vi "Drive States.vi"(10 "Drive Metrics in":T1) -> (2 "Drive Metrics out":T1)   [LabVIEW 2014]
uses:
  Drive Metrics.ctl
  Drive States.ctl
  Global Objects.vi
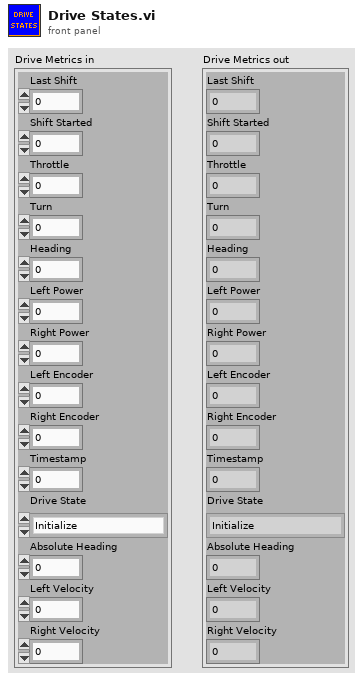
[diagram p1: front panel]
types:
  T1 = typedef "Drive Metrics.ctl" = cluster{"Last Shift":u32, "Shift Started":u32, "Throttle":dbl, "Turn":dbl, "Heading":dbl, "Left Power":dbl, "Right Power":dbl, "Left Encoder":dbl, "Right Encoder":dbl, "Timestamp":dbl, "Drive State":T2, "Absolute Heading":dbl, "Left Velocity":dbl, "Right Velocity":dbl}
  T2 = typedef "Drive States.ctl" = enum16{"Initialize", "Low Gear", "Up Shift Begin", "Up Shifting", "Up Shift Delay", "High Gear", "Down Shift Begin", "Down Shifting", "Down Shift Delay"}
  T3 = typedef "Configuration.ctl" = cluster{"Throttle Dead Zone":dbl, "Throttle Ramp Rate":dbl, "Turn Dead Zone":dbl, "Auton":cluster{"Motion Plan P":dbl, "Motion Plan I":dbl, "Motion Plan D":dbl}, "Auto Upshift Enabled":bool, "Upshift Min Throttle":dbl, "Upshift Min Velocity":dbl, "Min time before upshift":dbl, "Shift Throttle Detent":u32, "Min time before downshift":dbl, "Turn PID":cluster{"Motion Plan P":dbl, "Motion Plan I":dbl, "Motion Plan D":dbl}}
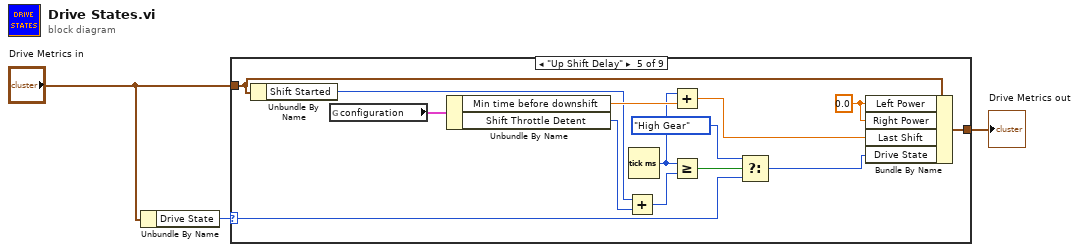
[diagram p0: block diagram]
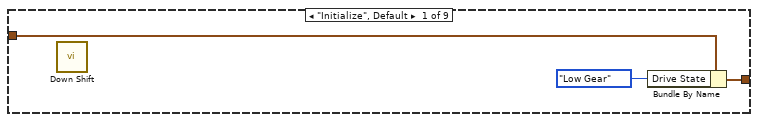
[diagram p2: hidden frame]
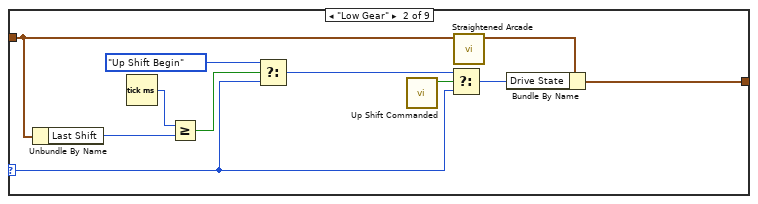
[diagram p3: hidden frame]
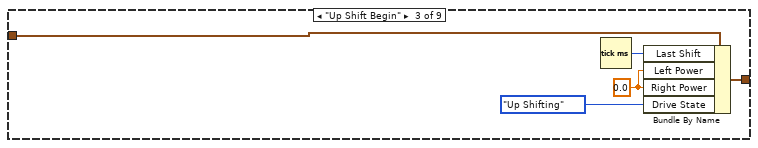
[diagram p4: hidden frame]
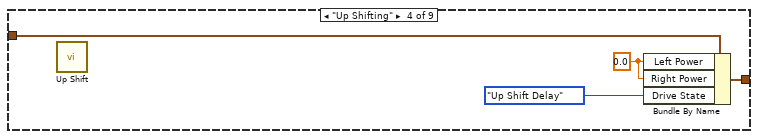
[diagram p5: hidden frame]
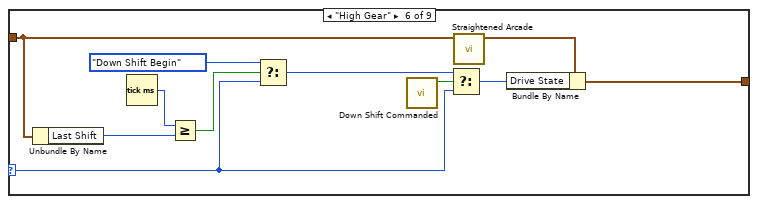
[diagram p6: hidden frame]
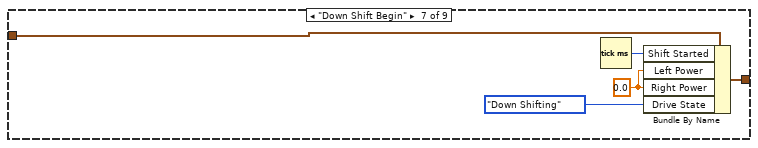
[diagram p7: hidden frame]
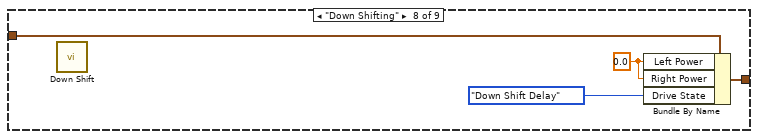
[diagram p8: hidden frame]
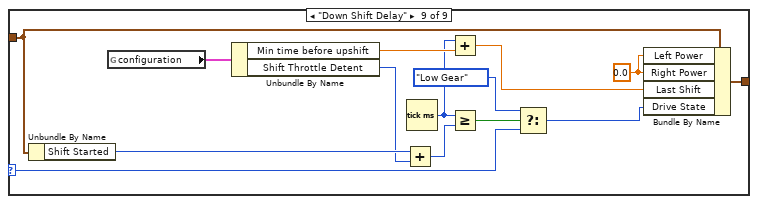
[diagram p9: hidden frame]
diagram:
  n1 = Unbundle By Name("Drive Metrics in") -> ("Drive State"=w1:T2)
  n2 = case shown="\"Up Shift Delay\"" w1 {
    selector: w1 -> [_ w12 _ _ w36 w47 _ _ w67]
    tunnel: "Drive Metrics in" -> [w6 w9 w22 w25 w29 w43 w56 w60 w63]
    tunnel: [w5 w8 w19 w24 w30 w42 w53 w58 w62] -> w3
    frame "Initialize", Default {
      n3 = call "Down Shift.vi"() -> ()  [unwired: 11 in, 1 out]
      n4 = Bundle By Name(cluster=w6, "Drive State"=Drive_States."Low Gear") -> (w5:T1)
    }
    frame "Low Gear" {
      n5 = Unbundle By Name(w9) -> ("Last Shift"=w15:u32)
      n6 = Tick Count (ms)() -> (millisecond timer value=w16:u32)
      n7 = Greater Or Equal?(x=w16, y=w15) -> (x >= y?=w14:bool)
      n8 = Select(t=Drive_States."Up Shift Begin", s=w14, f=w12) -> (s? t:f=w11:T2)
      n9 = call "Up Shift Commanded"() -> ("Up Shift Commanded"=w17:bool)  [unwired: 10 in, 1 out]
      n10 = Select(t=w11, s=w17, f=w12) -> (s? t:f=w7:T2)
      n11 = call "Straightened Arcade.vi"("Metrics In"=w9) -> ("Metrics Out"=w10:T1)  [unwired: 10 in]
      n12 = Bundle By Name(cluster=w10, "Drive State"=w7) -> (w8:T1)
    }
    frame "Up Shift Begin" {
      w20 = 0.0 ("Throttle")
      n13 = Tick Count (ms)() -> (millisecond timer value=w21:u32)
      n14 = Bundle By Name(cluster=w22, "Last Shift"=w21, "Left Power"=w20, "Right Power"=w20, "Drive State"=Drive_States."Up Shifting") -> (w19:T1)
    }
    frame "Up Shifting" {
      w26 = 0.0 ("Throttle")
      n15 = call "Up Shift.vi"() -> ()  [unwired: 11 in, 1 out]
      n16 = Bundle By Name(cluster=w25, "Left Power"=w26, "Right Power"=w26, "Drive State"=Drive_States."Up Shift Delay") -> (w24:T1)
    }
    frame "Up Shift Delay" {
      w34 = 0.0 ("Throttle")
      n17 = Unbundle By Name(w29) -> ("Shift Started"=w28:u32)
      n18 = global read "Global Objects.vi" "configuration"() -> (w40:T3)
      n19 = Unbundle By Name(w40) -> ("Min time before downshift"=w32:dbl, "Shift Throttle Detent"=w39:u32)
      n20 = Add(x=w28, y=w39) -> (x+y=w38:u32)
      n21 = Tick Count (ms)() -> (millisecond timer value=w31:u32)
      n22 = Add(x=w31, y=w32) -> (x+y=w33:dbl)
      n23 = Greater Or Equal?(x=w31, y=w38) -> (x >= y?=w37:bool)
      n24 = Select(t=Drive_States."High Gear", s=w37, f=w36) -> (s? t:f=w27:T2)
      n25 = Bundle By Name(cluster=w29, "Left Power"=w34, "Right Power"=w34, "Last Shift"=w33, "Drive State"=w27) -> (w30:T1)
    }
    frame "High Gear" {
      n26 = Unbundle By Name(w43) -> ("Last Shift"=w49:u32)
      n27 = Tick Count (ms)() -> (millisecond timer value=w50:u32)
      n28 = Greater Or Equal?(x=w50, y=w49) -> (x >= y?=w48:bool)
      n29 = Select(t=Drive_States."Down Shift Begin", s=w48, f=w47) -> (s? t:f=w45:T2)
      n30 = call "Down Shift Commanded.vi"() -> ("Down Shift Commanded"=w51:bool)  [unwired: 10 in, 1 out]
      n31 = Select(t=w45, s=w51, f=w47) -> (s? t:f=w41:T2)
      n32 = call "Straightened Arcade.vi"("Metrics In"=w43) -> ("Metrics Out"=w44:T1)  [unwired: 10 in]
      n33 = Bundle By Name(cluster=w44, "Drive State"=w41) -> (w42:T1)
    }
    frame "Down Shift Begin" {
      w54 = 0.0 ("Left Power")
      n34 = Tick Count (ms)() -> (millisecond timer value=w55:u32)
      n35 = Bundle By Name(cluster=w56, "Shift Started"=w55, "Left Power"=w54, "Right Power"=w54, "Drive State"=Drive_States."Down Shifting") -> (w53:T1)
    }
    frame "Down Shifting" {
      w59 = 0.0 ("Left Power")
      n36 = call "Down Shift.vi"() -> ()  [unwired: 11 in, 1 out]
      n37 = Bundle By Name(cluster=w60, "Left Power"=w59, "Right Power"=w59, "Drive State"=Drive_States."Down Shift Delay") -> (w58:T1)
    }
    frame "Down Shift Delay" {
      w74 = 0.0 ("Left Power")
      n38 = Unbundle By Name(w63) -> ("Shift Started"=w72:u32)
      n39 = global read "Global Objects.vi" "configuration"() -> (w73:T3)
      n40 = Unbundle By Name(w73) -> ("Min time before upshift"=w66:dbl, "Shift Throttle Detent"=w71:u32)
      n41 = Add(x=w72, y=w71) -> (x+y=w70:u32)
      n42 = Tick Count (ms)() -> (millisecond timer value=w65:u32)
      n43 = Add(x=w65, y=w66) -> (x+y=w64:dbl)
      n44 = Greater Or Equal?(x=w65, y=w70) -> (x >= y?=w69:bool)
      n45 = Select(t=Drive_States."Low Gear", s=w69, f=w67) -> (s? t:f=w61:T2)
      n46 = Bundle By Name(cluster=w63, "Left Power"=w74, "Right Power"=w74, "Last Shift"=w64, "Drive State"=w61) -> (w62:T1)
    }
  }
  "Drive Metrics out" <- w3
